vi "Get Stuct.vi"(11 "reference":refnum<vi>) -> (2 "Position":T1, 3 "Gen Refnum":refnum<vi>)   [LabVIEW 2015]
uses:
  <vilib>/Utility/miscctls.llb/LVPositionTypeDef.ctl
panel:
  out "Class Name":string
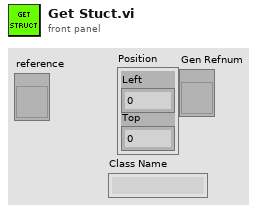
[diagram p1: front panel]
types:
  T1 = typedef "LVPositionTypeDef.ctl" = cluster{"Left":i32, "Top":i32}
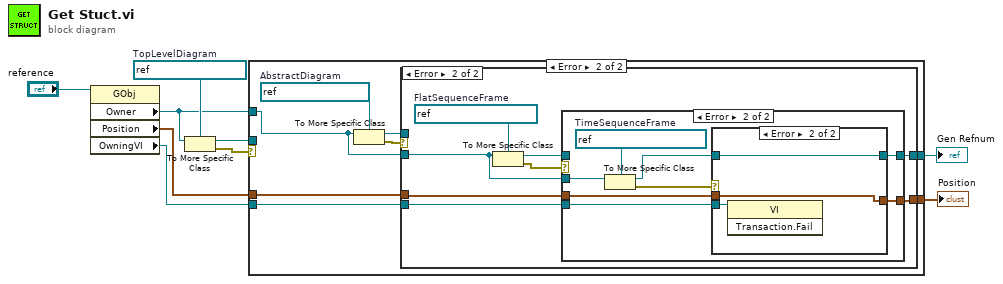
[diagram p0: block diagram]
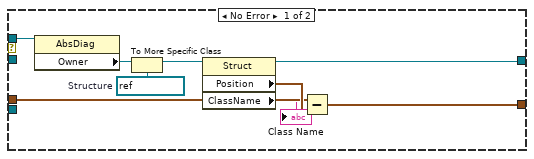
[diagram p3: hidden frame]
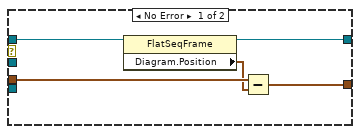
[diagram p4: hidden frame]
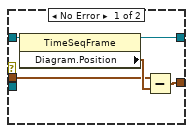
[diagram p5: hidden frame]
diagram:
  w9 = refnum<vi> refnum  # TopLevelDiagram
  n1 = property class="GObj"(reference="reference") -> ("Owner"=w2:refnum<vi>, "Position"=w4:T1, "OwningVI"=w1:refnum<vi>)  [unwired: 1 in, 2 out]
  n2 = To More Specific Class(target class=w9, reference=w2) -> (specific class reference=w5:refnum<vi>, error out=w8:errorcluster)  [unwired: 1 in]
  n3 = case shown="Error" w8 {
    tunnel: [w11 w17] -> w6
    tunnel: w4 -> [w11 w18]
    tunnel: [w10 w16] -> w3
    tunnel: w5 -> [w10 _]
    tunnel: w2 -> [_ w13]
    tunnel: w1 -> [_ w12]
    frame No Error {
    }
    frame Error {
      w19 = refnum<vi> refnum  # AbstractDiagram
      n4 = To More Specific Class(target class=w19, reference=w13) -> (specific class reference=w15:refnum<vi>, error out=w14:errorcluster)  [unwired: 1 in]
      n5 = case shown="Error" w14 {
        tunnel: w18 -> [w23 w32]
        tunnel: [w22 w31] -> w17
        tunnel: [w21 w30] -> w16
        tunnel: w15 -> [w28 _]
        tunnel: w13 -> [_ w33]
        tunnel: w12 -> [_ w29]
        frame No Error {
          w26 = refnum<vi> refnum  # Structure
          n6 = property class="AbsDiag"(reference=w28) -> ("Owner"=w27:refnum<vi>)  [unwired: 1 in, 2 out]
          n7 = To More Specific Class(target class=w26, reference=w27) -> (specific class reference=w24:refnum<vi>)  [unwired: 1 in, 1 out]
          n8 = property class="Struct"(reference=w24) -> (reference out=w21:refnum<vi>, "Position"=w25:T1, "ClassName"=→"Class Name":string)  [unwired: 1 in, 1 out]
          n9 = Subtract(x=w23, y=w25) -> (x-y=w22:T1)
        }
        frame Error {
          w35 = refnum<vi> refnum  # FlatSequenceFrame
          n10 = To More Specific Class(target class=w35, reference=w33) -> (specific class reference=w36:refnum<vi>, error out=w34:errorcluster)  [unwired: 1 in]
          n11 = case shown="Error" w34 {
            tunnel: w36 -> [w41 _]
            tunnel: w32 -> [w40 w46]
            tunnel: [w38 w44] -> w31
            tunnel: [w37 w43] -> w30
            tunnel: w33 -> [_ w48]
            tunnel: w29 -> [_ w42]
            frame No Error {
              n12 = property class="FlatSeqFrame"(reference=w41) -> (reference out=w37:refnum<vi>, "Diagram.Position"=w39:T1)  [unwired: 1 in, 1 out]
              n13 = Subtract(x=w40, y=w39) -> (x-y=w38:T1)
            }
            frame Error {
              w49 = refnum<vi> refnum  # TimeSequenceFrame
              n14 = To More Specific Class(target class=w49, reference=w48) -> (specific class reference=w45:refnum<vi>, error out=w47:errorcluster)  [unwired: 1 in]
              n15 = case shown="Error" w47 {
                tunnel: w46 -> [w53 w57]
                tunnel: w45 -> [w52 w56]
                tunnel: [w51 w57] -> w44
                tunnel: [w50 w56] -> w43
                tunnel: w42 -> [_ w55]
                frame No Error {
                  n16 = property class="TimeSeqFrame"(reference=w52) -> (reference out=w50:refnum<vi>, "Diagram.Position"=w54:T1)  [unwired: 1 in, 1 out]
                  n17 = Subtract(x=w53, y=w54) -> (x-y=w51:T1)
                }
                frame Error {
                  n18 = invoke class="VI" method="Transaction.Fail"(reference=w55) -> ()  [unwired: 2 in, 3 out]
                }
              }
            }
          }
        }
      }
    }
  }
  "Position" <- w6
  "Gen Refnum" <- w3
